vi "LauncherTest.vi"(8 "error in (no error)":errorcluster, 10 "SequncePath":string, 11 "UnitTestEngine in":refnum<class "UnitTestEngine.lvclass">) -> (0 "error out":errorcluster, 3 "UnitTestEngine out":refnum<class "UnitTestEngine.lvclass">)   [LabVIEW 2019, in "UnitTestEngine.lvlib" / "UnitTestEngine.lvclass"]
uses:
  UnitTestEngine.lvclass
  <vilib>/Utility/miscctls.llb/LVRowAndColumnTypeDef.ctl
  UnitTestEngine.lvclass/UnitTestEngine.ctl
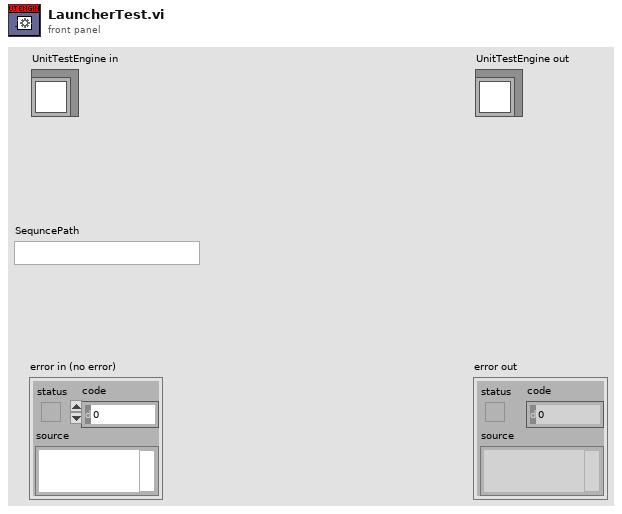
[diagram p1: front panel]
types:
  T1 = typedef "LVRowAndColumnTypeDef.ctl" = cluster{"Row":i32, "Column":i32}
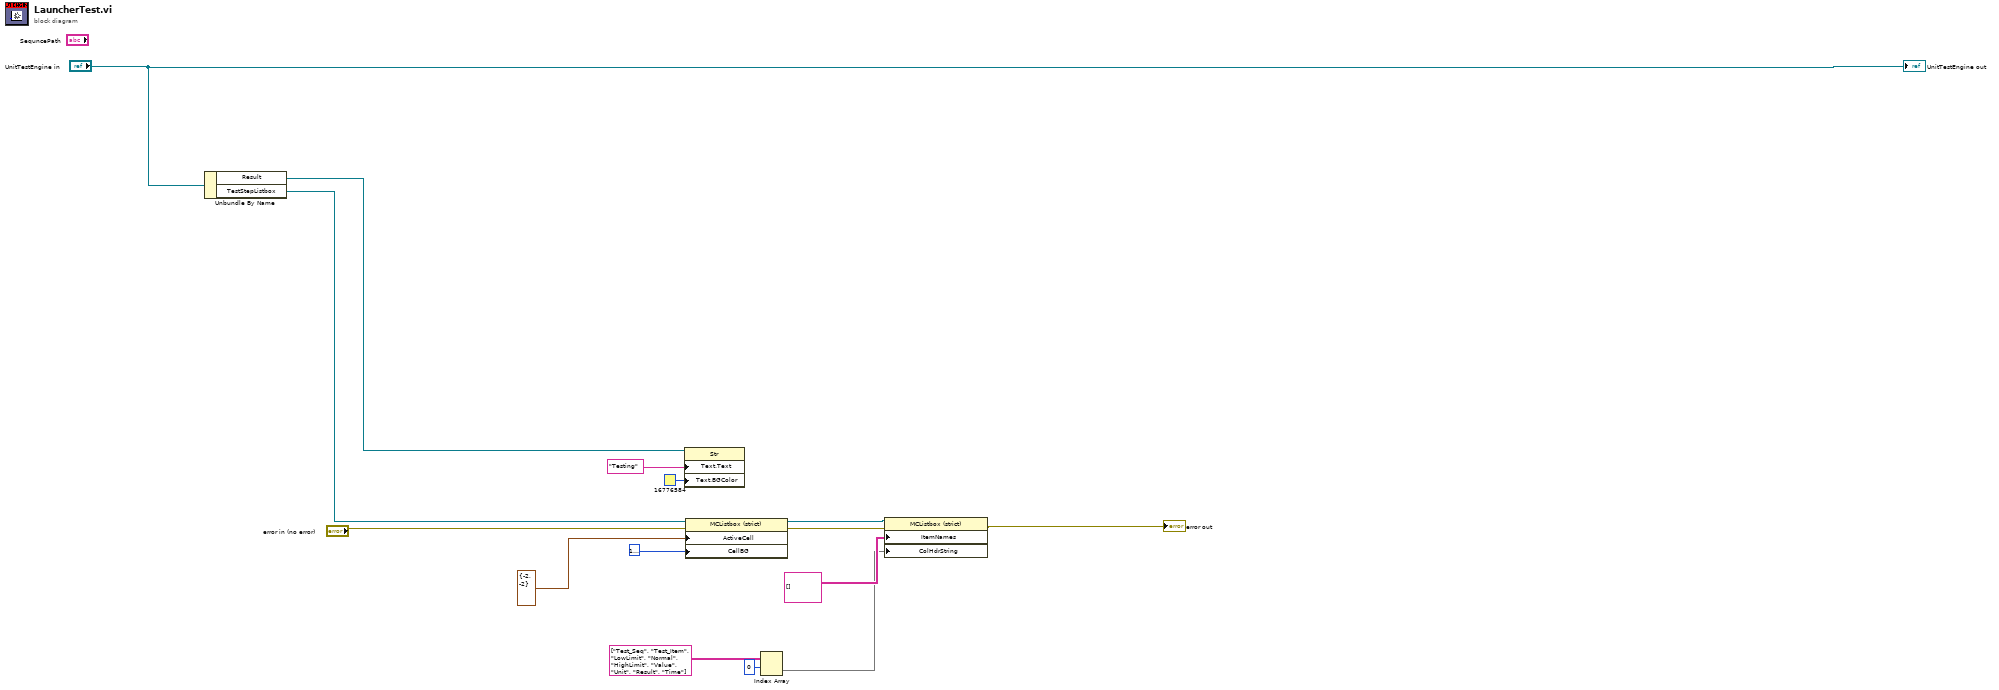
[diagram p0: block diagram]
diagram:
  n1 = Unbundle By Name("UnitTestEngine in") -> ("Result"=w6:refnum<vi>, "TestStepListbox"=w5:refnum<vi>)
  n2 = property class="Str"(reference=w6, "Text.Text"="Testing", "Text.BGColor"=u32 16776584 ("Text.Text Colors:Text Color")) -> ()  [unwired: 1 in, 2 out]
  n3 = property class="MCListbox (strict)"(reference=w5, error in="error in (no error)", "ActiveCell"=T1 {"Row"=-2, "Column"=-2} ("Active Cell:Active Cell"), "CellBG"=u32 16777225 ("Text.Text Colors:Text Color")) -> (reference out=w11:refnum<vi>, error out=w1:errorcluster)
  n4 = Index Array(array=string[][] [["Test_Seq", "Test_Item", "LowLimit", "Normal", "HighLimit", "Value", "Unit", "Result", "Time"]] ("ResultData"), index (row)=0 ("索引 (行)")) -> (element=w7:string[])  [unwired: 1 in]
  n5 = property class="MCListbox (strict)"(reference=w11, error in=w1, "ItemNames"=string[][] [] ("项名"), "ColHdrString"=w7) -> (error out=→"error out":errorcluster)  [unwired: 1 out]
  "UnitTestEngine out" <- "UnitTestEngine in"
